vi "Tree Tag String 2 RDB Receive Objects.vi"(11 "tag string":string) -> (2 "RDB Receive Objects":string caption="RDB Object Name", 3 "RDB Signalname":string)   [LabVIEW 2023, in "Vires VTD System Explorer.lvlib"]
uses:
  Vires VTD System Explorer.lvlib
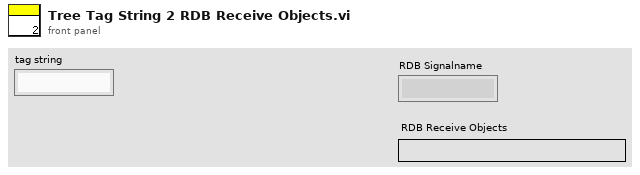
[diagram p1: front panel]
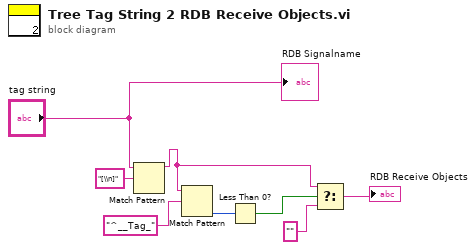
[diagram p0: block diagram]
diagram:
  n1 = Match Pattern(string="tag string", regular expression="[\\n]") -> (before substring=w3:string)  [unwired: 1 in, 3 out]
  n2 = Match Pattern(string=w3, regular expression="^__Tag_") -> (offset past match=w7:i32)  [unwired: 1 in, 3 out]
  n3 = Less Than 0?(x=w7) -> (x < 0?=w4:bool)
  n4 = Select(t=w3, s=w4, f="") -> (s? t:f=→"RDB Receive Objects":string)
  "RDB Signalname" <- "tag string"
